vi "PressureSensor.vi"(7 "Action":T4, 8 "error in (no error)":errorcluster, 10 "PressureScaler":dbl=1.0, 11 "AIDeviceRef":T1={"DevStatus"={"status"=FALSE, "code"=0, "source"=""}, "Analog Module"=enum."Analog Module 1", "Analog Channel"=enum."Invalid"}) -> (0 "error out":errorcluster, 3 "Pressure":dbl)   [LabVIEW 2013]
uses:
  PressureSensorAction.ctl
  <vilib>/Rock Robotics/WPI/AnalogChannel/WPI_AnalogChannelDevRef.ctl
  <vilib>/Rock Robotics/SystemInterfaces/Typedef/FPGA_TypedefAnalogModule.ctl
  <vilib>/Rock Robotics/SystemInterfaces/AI/FPGA_AIChannel.ctl
panel:
  in  "Samples Per Second":dbl=1000.0
  in  "AverageBits":u8=3
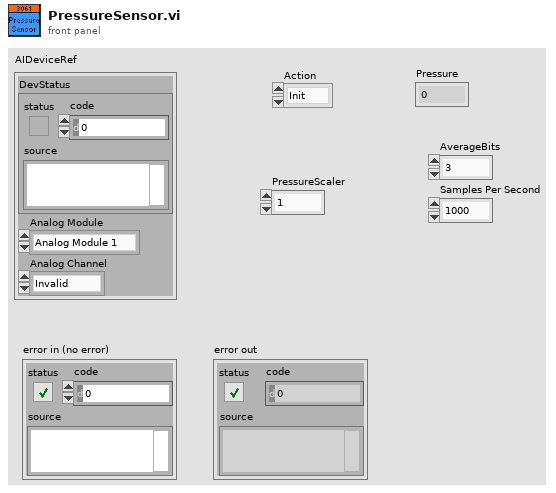
[diagram p1: front panel]
types:
  T1 = typedef "WPI_AnalogChannelDevRef.ctl" = cluster{"DevStatus":errorcluster, "Analog Module":T2, "Analog Channel":T3}
  T2 = typedef "FPGA_TypedefAnalogModule.ctl" = enum16{"Analog Module 1", "Analog Module 2"}
  T3 = typedef "FPGA_AIChannel.ctl" = enum8{"AI 1", "AI 2", "AI 3", "AI 4", "AI 5", "AI 6", "AI 7", "AI 8", "Invalid"}
  T4 = typedef "PressureSensorAction.ctl" = enum16{"Init", "ReadValue", "Disable"}
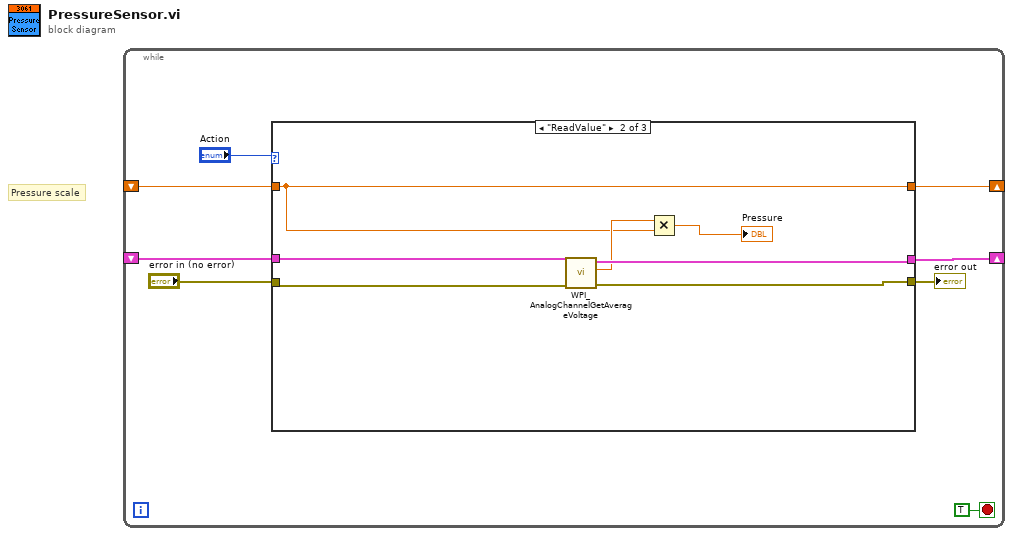
[diagram p0: block diagram]
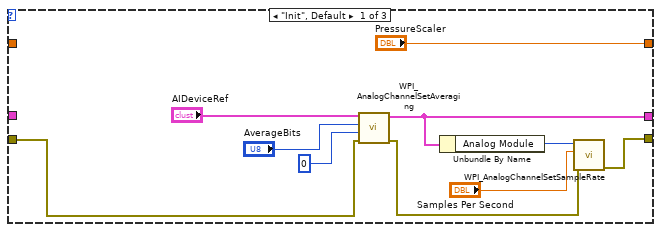
[diagram p2: hidden frame]
diagram:
  # "Pressure scale"
  n1 = while {
    shift-right: [w7] -> _
    shift-left: _ -> [w6]
    shift-right: [w2] -> _
    shift-left: _ -> [w1]
    stop <- TRUE stop-if-true
    n2 = case shown="\"ReadValue\"" "Action" {
      tunnel: [w17 w24 w28] -> w7
      tunnel: w6 -> [_ w25 w28]
      tunnel: "error in (no error)" -> [w12 w21 w27]
      tunnel: [w10 w20 w27] -> w4
      tunnel: ["PressureScaler" w19 w26] -> w2
      tunnel: w1 -> [_ w19 w26]
      frame "Init", Default {
        n3 = call <vilib>:"WPI_AnalogChannelSetAveraging.vi"("error in (no error)"=w12, "OversampleBits"=u8 0, "AverageBits"="AverageBits", "AIDeviceRef"="AIDeviceRef") -> ("error out"=w11:errorcluster, "AIDeviceRef"=w17:T1)  [unwired: 6 out]
        n4 = Unbundle By Name(w17) -> ("Analog Module"=w16:T2)
        n5 = call <vilib>:"WPI_AnalogChannelSetSampleRate.vi"("error in (no error)"=w11, "Samples Per Second"="Samples Per Second", "Analog Module (Module 1)"=w16) -> ("error out"=w10:errorcluster)  [unwired: 1 in, 7 out]
      }
      frame "ReadValue" {
        n6 = call <vilib>:"WPI_AnalogChannelGetAverageVoltage.vi"("error in (no error)"=w21, "AIDeviceRef"=w25) -> ("error out"=w20:errorcluster, "Voltage"=w23:dbl, "AIDeviceRef"=w24:T1)  [unwired: 7 out]
        n7 = Multiply(x=w23, y=w19) -> (x*y=→"Pressure":dbl)
      }
      frame "Disable" {
      }
    }
    "error out" <- w4
  }
